vi "MouseDown Response.vi"(4 "PlatMods":T1, 6 "Mods":cluster{"Double Click":bool, "Menu Key":bool}, 8 "error in (no error)":errorcluster, 9 "Button":u16, 10 "Coords":T2, 11 "Editor Handler in":refnum<class "Connector Editor Handler.lvclass">) -> (0 "error out":errorcluster, 3 "Editor Handler out":refnum<class "Connector Editor Handler.lvclass">)   [LabVIEW 2016, in "Connector Editor Handler.lvclass"]
uses:
  Connector Editor Handler.lvclass
  C:/Program Files (x86)/National Instruments/LabVIEW 2016/vi.lib/LIEF/Image Editor Handler/Image Editor Handler.lvclass
  <vilib>/Utility/miscctls.llb/LVPoint32TypeDef.ctl
  <vilib>/LIEF/Image Editor Handler/Image Editor Handler.lvclass/Image Editor Handler.ctl
  Connector Editor Handler.lvclass/Connector Editor Handler.ctl
  <vilib>/LIEF/Image Editor Handler/Write Selected.vi
  <vilib>/LIEF/Image Editor Handler/Read PictureRef.vi
  <vilib>/LIEF/Image Editor Handler/Read Shapes.vi
  <vilib>/LIEF/Image Editor Handler/Read Selected.vi
  <vilib>/LIEF/Image Editor Handler/Image Editor Handler.lvclass
  <vilib>/LIEF/Forms/Shape/Shape.lvclass
  <vilib>/LIEF/Forms/Link/Link.lvclass
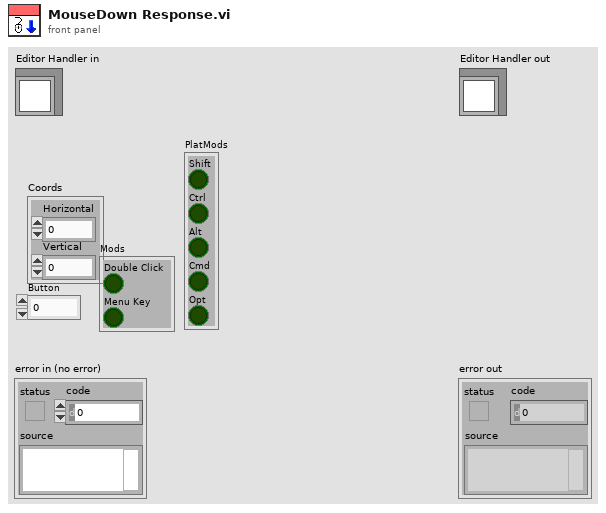
[diagram p1: front panel]
types:
  T1 = cluster{"Shift":bool, "Ctrl":bool, "Alt":bool, "Cmd":bool, "Opt":bool}
  T2 = typedef "LVPoint32TypeDef.ctl" = cluster{"Horizontal":i32, "Vertical":i32}
  T3 = typedef "LVPositionTypeDef.ctl" = cluster{"Left":i32, "Top":i32}
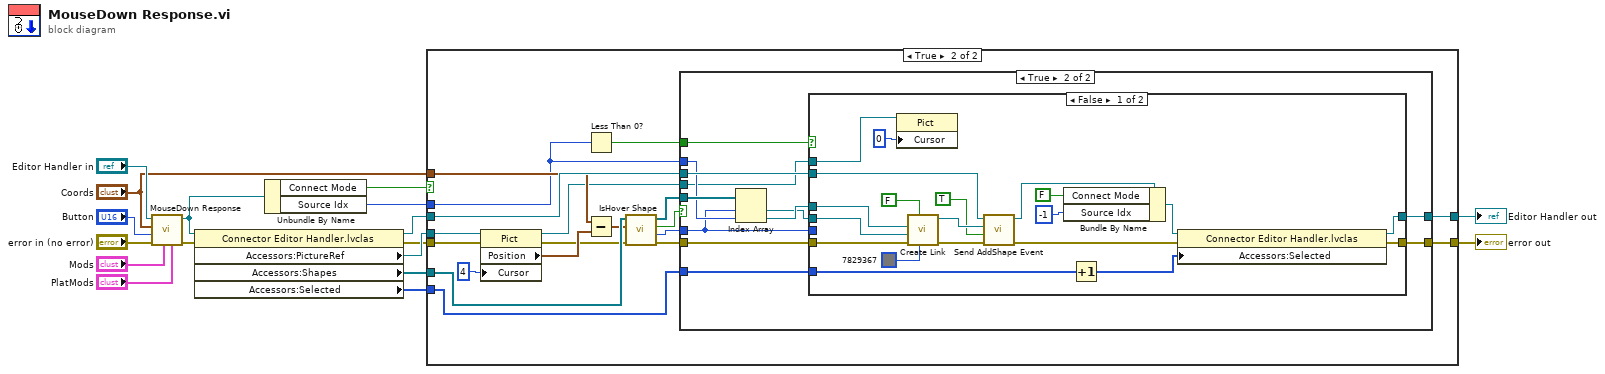
[diagram p0: block diagram]
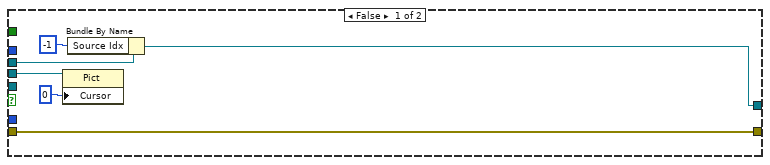
[diagram p3: hidden frame]
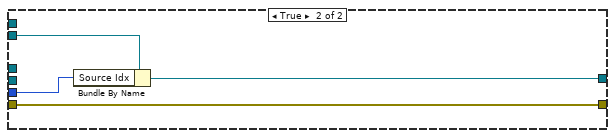
[diagram p4: hidden frame]
diagram:
  n1 = call-parent "MouseDown Response.vi"("PlatMods"="PlatMods", "Mods"="Mods", "error in (no error)"="error in (no error)", "Button"="Button", "Coords"="Coords", "Editor Handler in"="Editor Handler in") -> ("error out"=w5:errorcluster, "Editor Handler out"=w9:refnum<class "Connector Editor Handler.lvclass">)  [unwired: 4 in]
  n2 = property class="Connector Editor Handler.lvclas"(reference=w9, error in=w5) -> (reference out=w2:refnum<class "Connector Editor Handler.lvclass">, error out=w6:errorcluster, "Accessors:PictureRef"=w11:refnum<vi>, "Accessors:Shapes"=w12:refnum<data-value>[], "Accessors:Selected"=w1:i16[])
  n3 = Unbundle By Name(w9) -> ("Connect Mode"=w10:bool, "Source Idx"=w3:i32)
  n4 = case shown="True" w10 {
    tunnel: w12 -> [_ w38]
    tunnel: w11 -> [_ w37]
    tunnel: w2 -> [w19 w36]
    tunnel: [w19 w35] -> w8
    tunnel: "Coords" -> [_ w34]
    tunnel: w6 -> [w18 w33]
    tunnel: [w18 w20] -> w4
    tunnel: w3 -> [_ w26]
    tunnel: w1 -> [_ w24]
    frame False {
    }
    frame True {
      n5 = property class="Pict"(reference=w37, error in=w33, "Cursor"=4) -> (reference out=w22:refnum<vi>, error out=w30:errorcluster, "Position"=w32:T3)
      n6 = Less Than 0?(x=w26) -> (x < 0?=w25:bool)
      n7 = Subtract(x=w34, y=w32) -> (x-y=w31:T2)
      n8 = call <vilib>:"IsHover Shape.vi"("error in (no error)"=w30, "Coords"=w31, "Shape in"=w38) -> ("error out"=w21:errorcluster, "Node ID"=w27:i32, "Found?"=w29:bool, "Shape out"=w28:refnum<data-value>[])  [unwired: 3 in, 2 out]
      n9 = case shown="True" w29 {
        tunnel: w36 -> [w44 w56]
        tunnel: [w43 w55] -> w35
        tunnel: w26 -> [_ w52]
        tunnel: w25 -> [_ w54]
        tunnel: w28 -> [_ w53]
        tunnel: w27 -> [_ w49]
        tunnel: w24 -> [_ w48]
        tunnel: w22 -> [w40 w47]
        tunnel: w21 -> [w39 w46]
        tunnel: [w39 w45] -> w20
        frame False {
          n10 = property class="Pict"(reference=w40, "Cursor"=0) -> ()  [unwired: 1 in, 2 out]
          n11 = Bundle By Name(cluster=w44, "Source Idx"=-1) -> (w43:refnum<class "Connector Editor Handler.lvclass">)
        }
        frame True {
          n12 = Index Array(array=w53, index #1=w49, index #2=w52) -> (element #1=w50:refnum<data-value>, element #2=w51:refnum<data-value>)
          n13 = case shown="False" w54 {
            tunnel: w56 -> [w75 w80]
            tunnel: [w65 w79] -> w55
            tunnel: w50 -> [w76 _]
            tunnel: w51 -> [w72 _]
            tunnel: w49 -> [_ w78]
            tunnel: w48 -> [w67 _]
            tunnel: w47 -> [w63 _]
            tunnel: w46 -> [w58 w77]
            tunnel: [w57 w77] -> w45
            frame False {
              n14 = property class="Pict"(reference=w63, "Cursor"=0) -> ()  [unwired: 1 in, 2 out]
              n15 = call <vilib>:"Create Link.vi"("Color"=u32 7829367, "Selectable"=FALSE, "error in (no error)"=w58, "Destination"=w76, "Source"=w72) -> ("error out"=w59:errorcluster, "Link Reference"=w74:refnum<data-value>)  [unwired: 5 in]
              n16 = call <vilib>:"Send AddShape Event.vi"("error in (no error)"=w59, "Backward"=TRUE, "New Shape Reference"=w74, "Editor Handler in"=w75) -> ("error out"=w60:errorcluster, "Editor Handler out"=w73:refnum<class "Connector Editor Handler.lvclass">)  [unwired: 6 in]
              n17 = Bundle By Name(cluster=w73, "Connect Mode"=FALSE, "Source Idx"=-1) -> (w68:refnum<class "Connector Editor Handler.lvclass">)
              n18 = Increment(x=w67) -> (x+1=w66:i16[])
              n19 = property class="Connector Editor Handler.lvclas"(reference=w68, error in=w60, "Accessors:Selected"=w66) -> (reference out=w65:refnum<class "Connector Editor Handler.lvclass">, error out=w57:errorcluster)
            }
            frame True {
              n20 = Bundle By Name(cluster=w80, "Source Idx"=w78) -> (w79:refnum<class "Connector Editor Handler.lvclass">)
            }
          }
        }
      }
    }
  }
  "error out" <- w4
  "Editor Handler out" <- w8
